vi "Check coord input.vi"(10 "coordIn":string, 11 "RA=T, default: F=DEC":bool) -> (2 "coordOut":string, 3 "valid":bool)   [LabVIEW 2018]
uses:
  <vilib>/regexp/Match Regular Expression.xnode
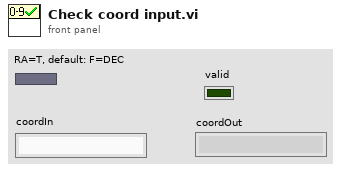
[diagram p1: front panel]
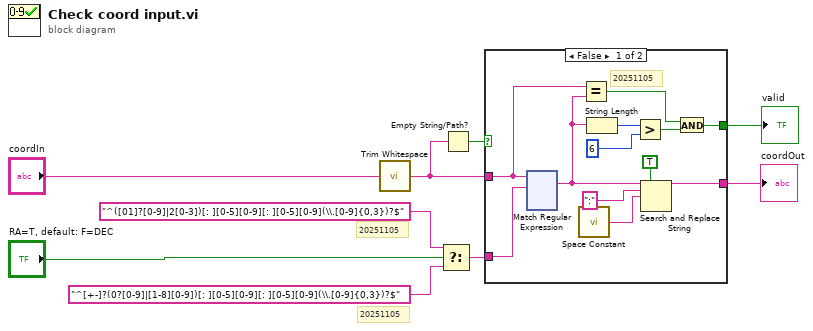
[diagram p0: block diagram]
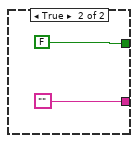
[diagram p2: hidden frame]
diagram:
  # "20251105"
  # "20251105"
  n1 = call <vilib>:"Trim Whitespace.vi"("string"="coordIn") -> ("trimmed string"=w8:string)  [unwired: 1 in]
  n2 = Select(t="^([01]?[0-9]|2[0-3])[: ][0-5][0-9][: ][0-5][0-9](\\.[0-9]{0,3})?$" ("Regular Expression"), s="RA=T, default: F=DEC", f="^[+-]?(0?[0-9]|[1-8][0-9])[: ][0-5][0-9][: ][0-5][0-9](\\.[0-9]{0,3})?$" ("Regular Expression")) -> (s? t:f=w2:string)
  n3 = Empty String/Path?(string/path=w8) -> (empty?=w7:bool)
  n4 = case shown="False" w7 {
    tunnel: w8 -> [w12 _]
    tunnel: w2 -> [w21 _]
    tunnel: [w13 FALSE] -> w6
    tunnel: [w14 ""] -> w1
    frame False {
      # "20251105"
      n5 = xnode "Match Regular Expression"("input string"=w12, "regular expression"=w21) -> ("whole match"=w11:string)  [unwired: 4 in, 4 out]
      n6 = call <vilib>:"Space Constant.vi"() -> ("String"=w16:string)
      n7 = Equal?(x=w12, y=w11) -> (x = y?=w10:bool)
      n8 = String Length(string=w11) -> (length=w19:i32)
      n9 = Greater?(x=w19, y=6) -> (0:w20:bool)
      n10 = Search and Replace String(replace all?=TRUE ("replace all? (F)"), input string=w11, search string=":", replace string=w16) -> (result string=w14:string)  [unwired: 4 in, 3 out]
      n11 = And(x=w10, y=w20) -> (x .and. y?=w13:bool)
    }
    frame True {
    }
  }
  "valid" <- w6
  "coordOut" <- w1
